vi "Get Count (Global).vi"() -> (3 "Count":u32)   [LabVIEW 2014, in "Device Configuration.lvclass"]
uses:
  Device Configuration/Device Configuration.lvclass
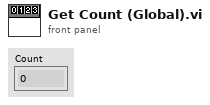
[diagram p1: front panel]
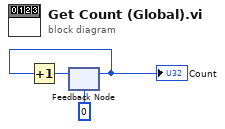
[diagram p0: block diagram]
diagram:
  n1 = feedback #1(u32 0) -> (w3:u32)
  "Count" <- w3
  n2 = Increment(x=w3) -> (x+1=w1:u32)
  n3 = feedback-in #1(w1) -> ()
